vi "Innitialize Shift Register.vi"() -> ()   [LabVIEW 2015]
panel:
  out "Data":u32
  out "Iterasi":u32
  out "Out":u32
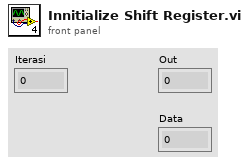
[diagram p1: front panel]
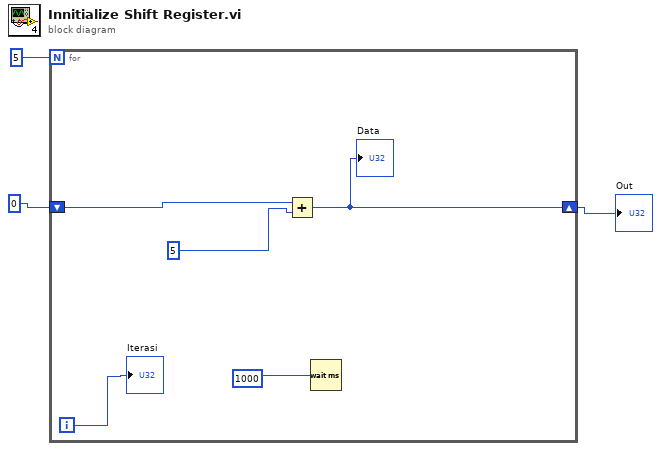
[diagram p0: block diagram]
diagram:
  n1 = for {
    N: 5 -> [_]
    shift-right: [w4] -> w3
    shift-left: 0 -> [w5]
    i -> [w6]
    n2 = Add(x=w5, y=5) -> (x+y=w4:i32)
    "Data" <- w4
    n3 = Wait (ms)(milliseconds to wait=1000) -> ()  [unwired: 1 out]
    "Iterasi" <- w6
  }
  "Out" <- w3
